vi "Test_BL_Profile.vi"() -> ()   [LabVIEW 2010]
panel:
  out "XY Graph":cluster{i32[], dbl[]}(graph)
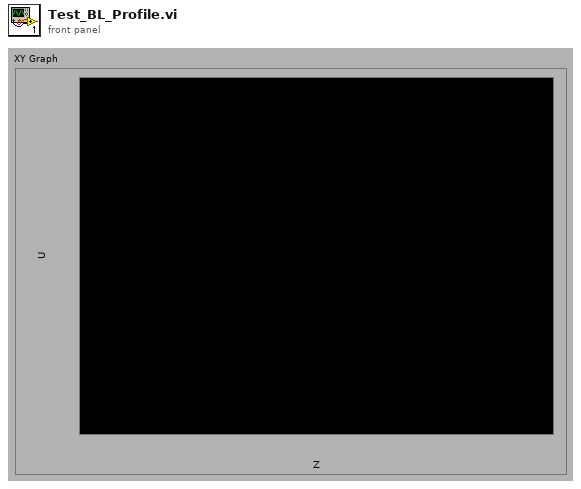
[diagram p1: front panel]
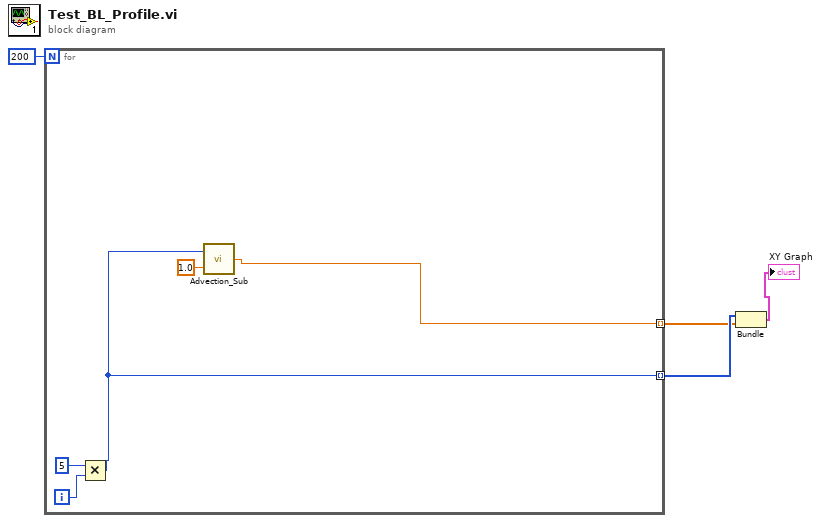
[diagram p0: block diagram]
diagram:
  n1 = for {
    N: 200 -> [_]
    tunnel: [w6] -> w3 mode=indexing
    tunnel: [w5] -> w2 mode=indexing
    i -> [w9]
    n2 = Multiply(x=5, y=w9) -> (x*y=w6:i32)
    n3 = call "Advection_Sub.vi"("Uref"=1.0, "Z"=w6) -> ("U m/s"=w5:dbl)
  }
  n4 = Bundle(w3, w2) -> (→"XY Graph":cluster{i32[], dbl[]})  [unwired: 1 in]
